vi "MC5e Build_Squad_Listbox.vi"(8 "error in (no error)":errorcluster, 11 "Squad Summary Ref":refnum<vi>) -> (0 "error out":errorcluster)   [LabVIEW 2020]
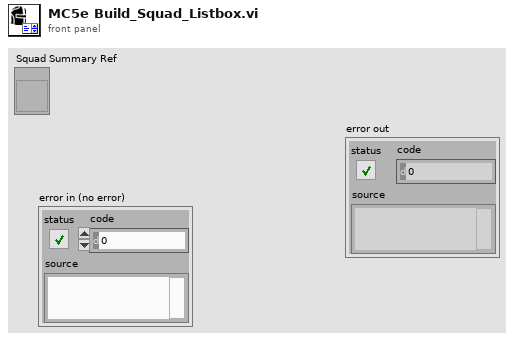
[diagram p1: front panel]
types:
  T1 = typedef "MC5e Squad_Info.ctl" = cluster{"Squad Name":string, "# Soldiers":u16, "Battle Rating":u16, "Flying":bool, "Mounted":bool, "Speed":u16, "Range":u16, "Morale":i32, "Max Endurance":u16, "Current Endurance":i32, "Size":T2, "Space Taken":u16, "Difficult Terrain":i32[], "CR":u16, "Special / Notes":string}
  T2 = typedef "MC5e Size_Categories.ctl" = enum16{"Tiny", "Small", "Medium", "Large", "Huge", "Gargantuan"}
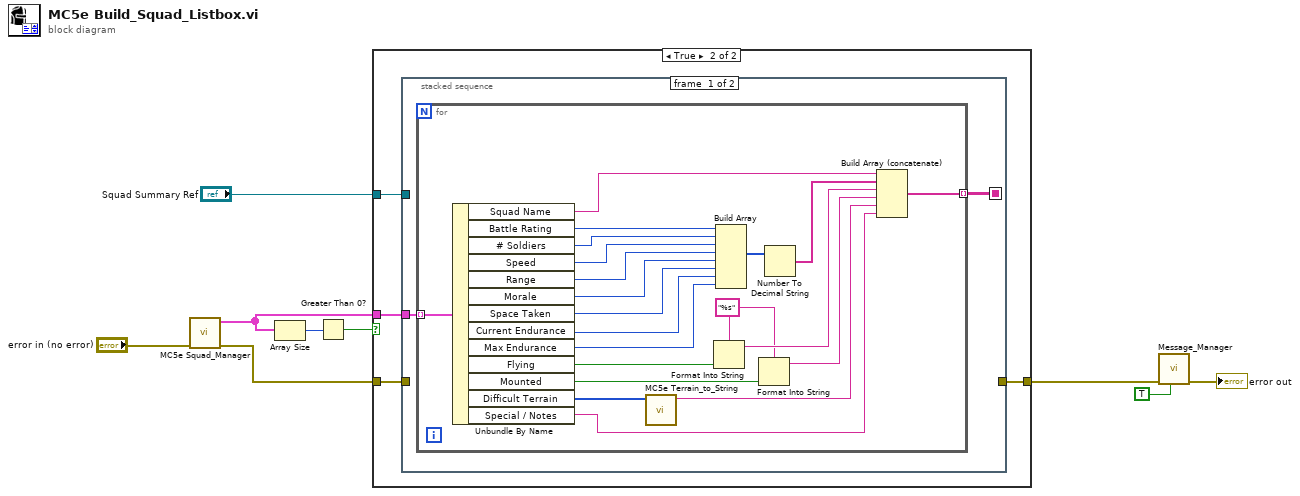
[diagram p0: block diagram]
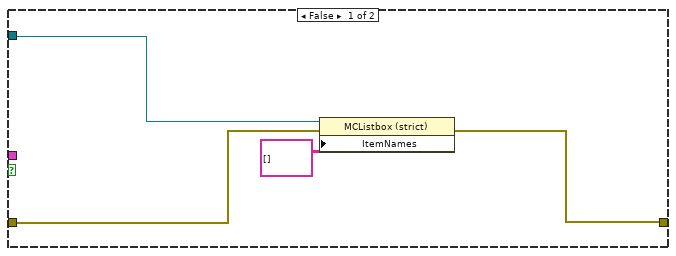
[diagram p2: hidden frame]
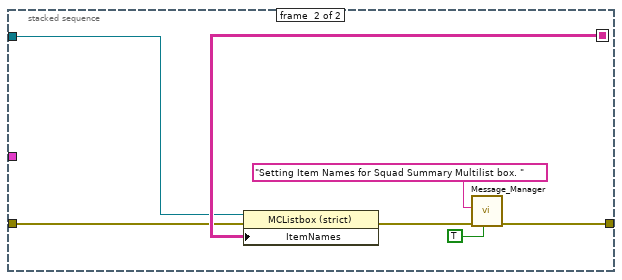
[diagram p3: hidden frame]
diagram:
  n1 = call "MC5e Squad_Manager.vi"("error in"="error in (no error)") -> ("error out"=w9:errorcluster, "All Squads Out"=w1:T1[])  [unwired: 7 in, 2 out]
  n2 = Array Size(array=w1) -> (size(s)=w2:i32)
  n3 = Greater Than 0?(x=w2) -> (x > 0?=w7:bool)
  n4 = case shown="True" w7 {
    tunnel: w9 -> [w11 w17]
    tunnel: w1 -> [_ w16]
    tunnel: [w10 w15] -> w5
    tunnel: "Squad Summary Ref" -> [w12 w14]
    frame False {
      n5 = property class="MCListbox (strict)"(reference=w12, error in=w11, "ItemNames"=string[][] [] ("Item Names")) -> (error out=w10:errorcluster)  [unwired: 1 out]
    }
    frame True {
      n6 = stacked-sequence {
        seq-local: [w18 _] -> [_ w47]
        tunnel: w17 -> [_ w46]
        tunnel: w16 -> [w19 _]
        tunnel: [_ w42] -> w15
        tunnel: w14 -> [_ w45]
        frame #0 {
          n7 = for {
            tunnel: w19 -> [w40] mode=indexing
            tunnel: [w26] -> w18 mode=indexing
            w25 = "%s" ("format string")
            n8 = Unbundle By Name(w40) -> ("Squad Name"=w20:string, "Battle Rating"=w21:u16, "# Soldiers"=w23:u16, "Speed"=w39:u16, "Range"=w38:u16, "Morale"=w37:i32, "Space Taken"=w22:u16, "Current Endurance"=w36:i32, "Max Endurance"=w35:u16, "Flying"=w33:bool, "Mounted"=w32:bool, "Difficult Terrain"=w31:i32[], "Special / Notes"=w27:string)
            n9 = call "MC5e Terrain_to_String.vi"("Difficult Terrain"=w31) -> ("Difficult Terrain String"=w28:string)  [unwired: 10 in]
            n10 = Format Into String(format string=w25, w33) -> (resulting string=w29:string)  [unwired: 2 in, 1 out]
            n11 = Build Array(w21, w23, w39, w38, w37, w22, w36, w35) -> (w34:i32[])
            n12 = Format Into String(format string=w25, w32) -> (resulting string=w24:string)  [unwired: 2 in, 1 out]
            n13 = Number To Decimal String(number=w34) -> (decimal integer string=w30:string[])  [unwired: 1 in]
            n14 = Build Array (concatenate)(w20, w30, w29, w24, w28, w27) -> (w26:string[])
          }
        }
        frame #1 {
          n15 = property class="MCListbox (strict)"(reference=w45, error in=w46, "ItemNames"=w47) -> (error out=w43:errorcluster)  [unwired: 1 out]
          n16 = call "Message_Manager.vi"("Log only on Err (F)"=TRUE ("Log only on Err"), "error in"=w43, "New Entry"="Setting Item Names for Squad Summary Multilist box. ") -> ("error out"=w42:errorcluster)  [unwired: 4 in, 4 out]
        }
      }
    }
  }
  n17 = call "Message_Manager.vi"("Log only on Err (F)"=TRUE ("Log only on Err"), "error in"=w5) -> ("error out"=→"error out":errorcluster)  [unwired: 5 in, 4 out]
